vi "VIn SMU.vi"(7 "Current Limit":dbl, 8 "error in (no error)":errorcluster, 9 "Voltage Level":dbl, 10 "Vin SMU Channel":string, 11 "IVI Refnum in":refnum<k15>) -> (0 "error out":errorcluster, 2 "Current Measurement":dbl caption="Vin SMU Current", 3 "Voltage Measurement":dbl caption="Vin SMU Voltage")   [LabVIEW 2021]
uses:
  <instrlib>/niDCPower/nidcpower.llb/niDCPower Source Mode.ctl
  <instrlib>/niDCPower/nidcpower.llb/niDCPower Output Function.ctl
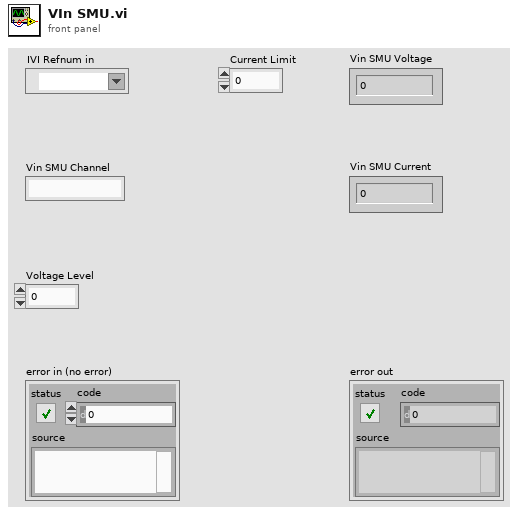
[diagram p1: front panel]
types:
  T1 = typedef "niDCPower Output Function.ctl" = i32
  T2 = typedef "niDCPower Source Mode.ctl" = i32
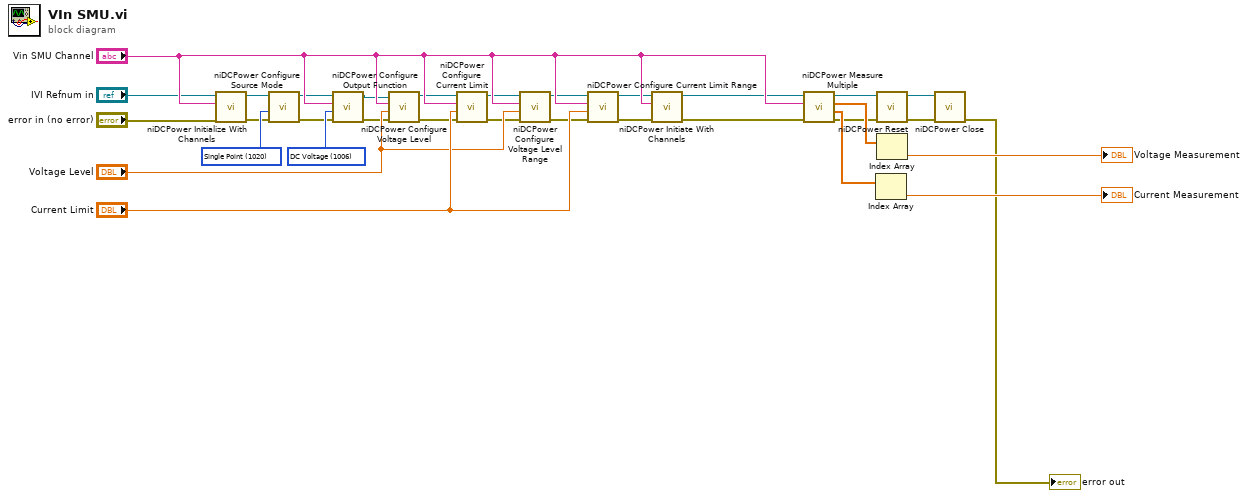
[diagram p0: block diagram]
diagram:
  w23 = T1 1006 items=["DC Voltage"=1006, "DC Current"=1007, "Pulse Voltage"=1049, "Pulse Current"=1050] ("output function")
  w10 = T2 1020 items=["Single Point"=1020, "Sequence"=1021] ("source mode")
  n1 = call <instrlib>:"niDCPower Initialize With Channels.vi"("error in (no error)"="error in (no error)", "channels"="Vin SMU Channel", "resource name"="IVI Refnum in") -> ("error out"=w6:errorcluster, "instrument handle out"=w7:refnum<k15>)  [unwired: 2 in, 5 out]
  n2 = call <instrlib>:"niDCPower Configure Source Mode.vi"("error in (no error)"=w6, "source mode"=w10, "instrument handle"=w7) -> ("error out"=w8:errorcluster, "instrument handle out"=w9:refnum<k15>)  [unwired: 7 out]
  n3 = call <instrlib>:"niDCPower Configure Output Function.vi"("error in (no error)"=w8, "output function"=w23, "channel name"="Vin SMU Channel", "instrument handle"=w9) -> ("error out"=w22:errorcluster, "instrument handle out"=w21:refnum<k15>)  [unwired: 6 out]
  n4 = call <instrlib>:"niDCPower Configure Voltage Level.vi"("error in (no error)"=w22, "voltage level"="Voltage Level", "channel name"="Vin SMU Channel", "instrument handle"=w21) -> ("error out"=w3:errorcluster, "instrument handle out"=w2:refnum<k15>)  [unwired: 6 out]
  n5 = call <instrlib>:"niDCPower Configure Current Limit.vi"("error in (no error)"=w3, "current limit"="Current Limit", "channel name"="Vin SMU Channel", "instrument handle"=w2) -> ("error out"=w11:errorcluster, "instrument handle out"=w12:refnum<k15>)  [unwired: 1 in, 5 out]
  n6 = call <instrlib>:"niDCPower Configure Voltage Level Range.vi"("error in (no error)"=w11, "voltage level range"="Voltage Level", "channel name"="Vin SMU Channel", "instrument handle"=w12) -> ("error out"=w13:errorcluster, "instrument handle out"=w14:refnum<k15>)  [unwired: 6 out]
  n7 = call <instrlib>:"niDCPower Configure Current Limit Range.vi"("error in (no error)"=w13, "current limit range"="Current Limit", "channel name"="Vin SMU Channel", "instrument handle"=w14) -> ("error out"=w18:errorcluster, "instrument handle out"=w17:refnum<k15>)  [unwired: 6 out]
  n8 = call <instrlib>:"niDCPower Initiate With Channels.vi"("error in (no error)"=w18, "channel name"="Vin SMU Channel", "instrument handle"=w17) -> ("error out"=w20:errorcluster, "instrument handle out"=w19:refnum<k15>)  [unwired: 7 in]
  n9 = call <instrlib>:"niDCPower Measure Multiple.vi"("error in (no error)"=w20, "channel name"="Vin SMU Channel", "instrument handle"=w19) -> ("error out"=w16:errorcluster, "current measurements"=w25:dbl[], "voltage measurements"=w27:dbl[], "instrument handle out"=w15:refnum<k15>)  [unwired: 5 out]
  n10 = Index Array(array=w25) -> (element=→"Current Measurement":dbl)  [unwired: 1 in]
  n11 = call <instrlib>:"niDCPower Reset.vi"("error in (no error)"=w16, "instrument handle"=w15) -> ("error out"=w5:errorcluster, "instrument handle out"=w4:refnum<k15>)  [unwired: 2 in, 6 out]
  n12 = Index Array(array=w27) -> (element=→"Voltage Measurement":dbl)  [unwired: 1 in]
  n13 = call <instrlib>:"niDCPower Close.vi"("error in (no error)"=w5, "instrument handle"=w4) -> ("error out"=→"error out":errorcluster)  [unwired: 9 out]
